vi "Get Node Data (DBL).vi"(3 "element id":i32, 6 "Attribute?(F=Entity)":bool, 7 "format string":string, 8 "error in":errorcluster, 9 "Default Value (0.0)":dbl, 10 "Attribute Name":string, 11 "xml":T1) -> (0 "error out":errorcluster, 1 "Attribute Value":dbl, 2 "found?":bool)   [LabVIEW 2013]
doc: "Returns the <B>Data Value</B> (text or cdata-section) of <B>Node</B>. If none is found, <B>Default Value</B> will be used."
uses:
  Fast Parser/XML Structure - Cluster.ctl
  Fast Parser/XML Tag Type - Enum.ctl
panel:
  # "Copyright © 2006 James Kring, Inc. All rights reserved.\n\nAuthor: Jim Kring <jim.kring@jameskring.com>\n\nThis library is provided \"AS IS\" , WITHOUT WARRANTIES OR \nCONDITIONS OF ANY KIND, either express or implied.\n\nJames Kring, Inc. -- http://www.jameskring.com"
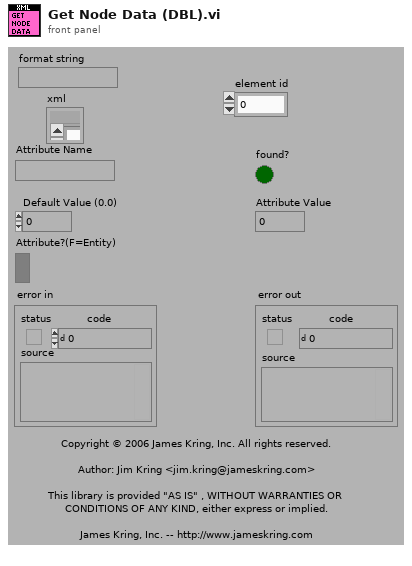
[diagram p1: front panel]
types:
  T1 = typedef "XML Structure - Cluster.ctl" = cluster{"tags":string[], "tag names":string[], "tag type":T2[], "offset":i32[], "close tag index":i32[], "xml":string, "Children":cluster{"children":i32[]}[], "parent index":i32[]}
  T2 = typedef "XML Tag Type - Enum.ctl" = enum16{"start tag", "empty tag", "end tag"}
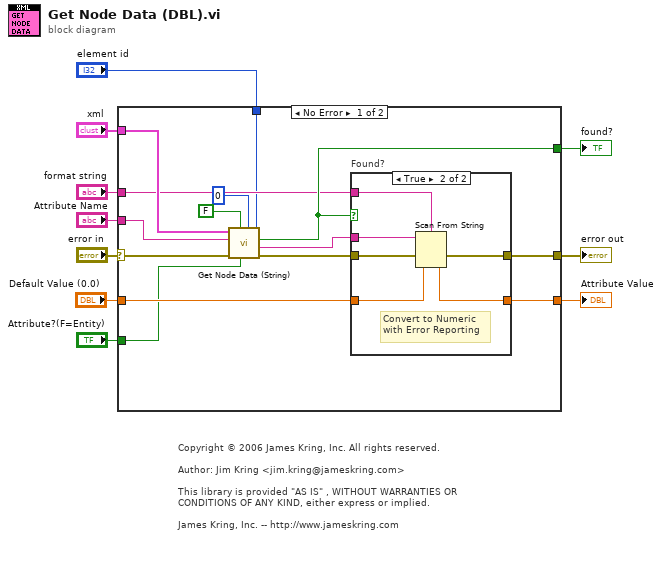
[diagram p0: block diagram]
diagram:
  # "Copyright © 2006 James Kring, Inc. All rights reserved.\n\nAuthor: Jim Kring <jim.kring@jameskring.com>\n\nThis library is provided \"AS IS\" , WITHOUT WARRANTIES OR \nCONDITIONS OF ANY KIND, either express or implied.\n\nJames Kring, Inc. -- http://www.jameskring.com"
  n1 = case shown="No Error" "error in" {
    selector: "error in" -> [w23 w34]
    tunnel: "xml" -> [w24 _]
    tunnel: [w17 w33] -> w9
    tunnel: [w21 w34] -> w10
    tunnel: [w20 _] -> w6
    tunnel: "Default Value (0.0)" -> [w18 w33]
    tunnel: "format string" -> [w16 _]
    tunnel: "Attribute?(F=Entity)" -> [w14 _]
    tunnel: "Attribute Name" -> [w15 _]
    tunnel: "element id" -> [w11 _]
    frame No Error {
      n2 = call "Get Node Data (String).vi"("element id"=w11, "level"=0, "Attribute? (F=Entity)"=w14, "contains raw xml"=FALSE, "error in (no error)"=w23, "Attribute Name"=w15, "xml"=w24) -> ("error out"=w22:errorcluster, "Data Value"=w19:string, "found?"=w20:bool)  [unwired: 2 in]
      n3 = case "Found?" shown="True" w20 {
        tunnel: w22 -> [w25 w29]
        tunnel: [w25 w28] -> w21
        tunnel: w19 -> [_ w32]
        tunnel: w18 -> [w26 w31]
        tunnel: [w26 w30] -> w17
        tunnel: w16 -> [_ w27]
        frame False {
        }
        frame True {
          # "Convert to Numeric\nwith Error Reporting"
          n4 = Scan From String(format string=w27, input string=w32, error in=w29, default 1=w31) -> (error out=w28:errorcluster, output 1=w30:dbl)  [unwired: 1 in, 2 out]
        }
      }
    }
    frame Error {
    }
  }
  "error out" <- w10
  "Attribute Value" <- w9
  "found?" <- w6
